vi "Fetch Multiple Record Multiple Channel (Wfm).vi"(5 "FIFO Type":T1=enum."Fast FIFO", 7 "Timeout (s)":i32=5, 8 "error in":errorcluster, 10 "Records to Fetch":i32, 11 "FPGA VI Reference In":refnum<k20>) -> (0 "error out":errorcluster, 2 "Acquired Data":waveform(dbl)[](array[waveform]), 3 "FPGA VI Reference Out":refnum<k20>, 4 "Elements Remaining":u32)   [LabVIEW 2012]
uses:
  <userlib>/FlexRIO Host Library/FlexRIO Host API/Acquire/FIFO Type.ctl
  <userlib>/FlexRIO Host Library/FlexRIO Host API/Acquire/Fetch/Fetch Acquired Data (I16).vi
  <vilib>/Utility/error.llb/Error Cluster From Error Code.vi
  <vilib>/rvi/errors/niLvFpgaAdjustHostInterfaceError.vi
  <vilib>/rvi/interface/nirviReadWriteControl/nirviReadWriteControl.xnode
  NiFpgaLv.dll
  <vilib>/rvi/interface/Simulation/niFpgaSimulationCallBeginRW.vi
  <userlib>/FlexRIO Host Library/FlexRIO Host Library (User).lvlib
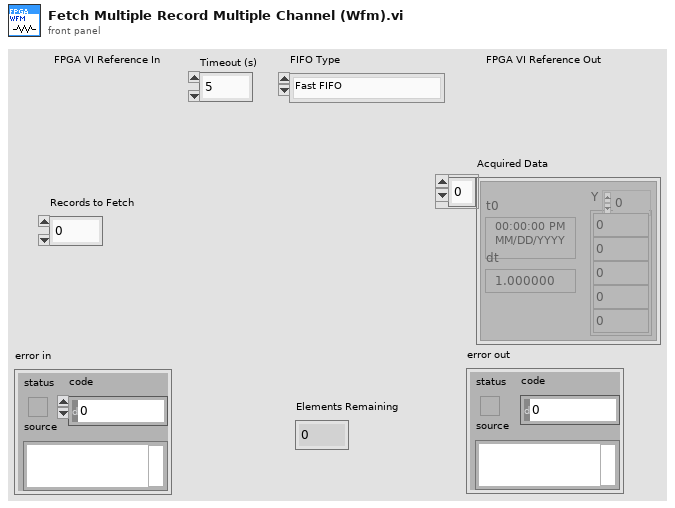
[diagram p1: front panel]
types:
  T1 = typedef "FIFO Type.ctl" = enum16{"FPGA to Host FIFO (U64)", "Generic", "FPGA to Host FIFO (U32)", "Fast FIFO"}
  T2 = cluster{"Load Record Parameters?":bool, "Pre Trigger Samples":u16, "Samples per Record":u16, "Trigger Hold Off":u16, "Record Count":u16}
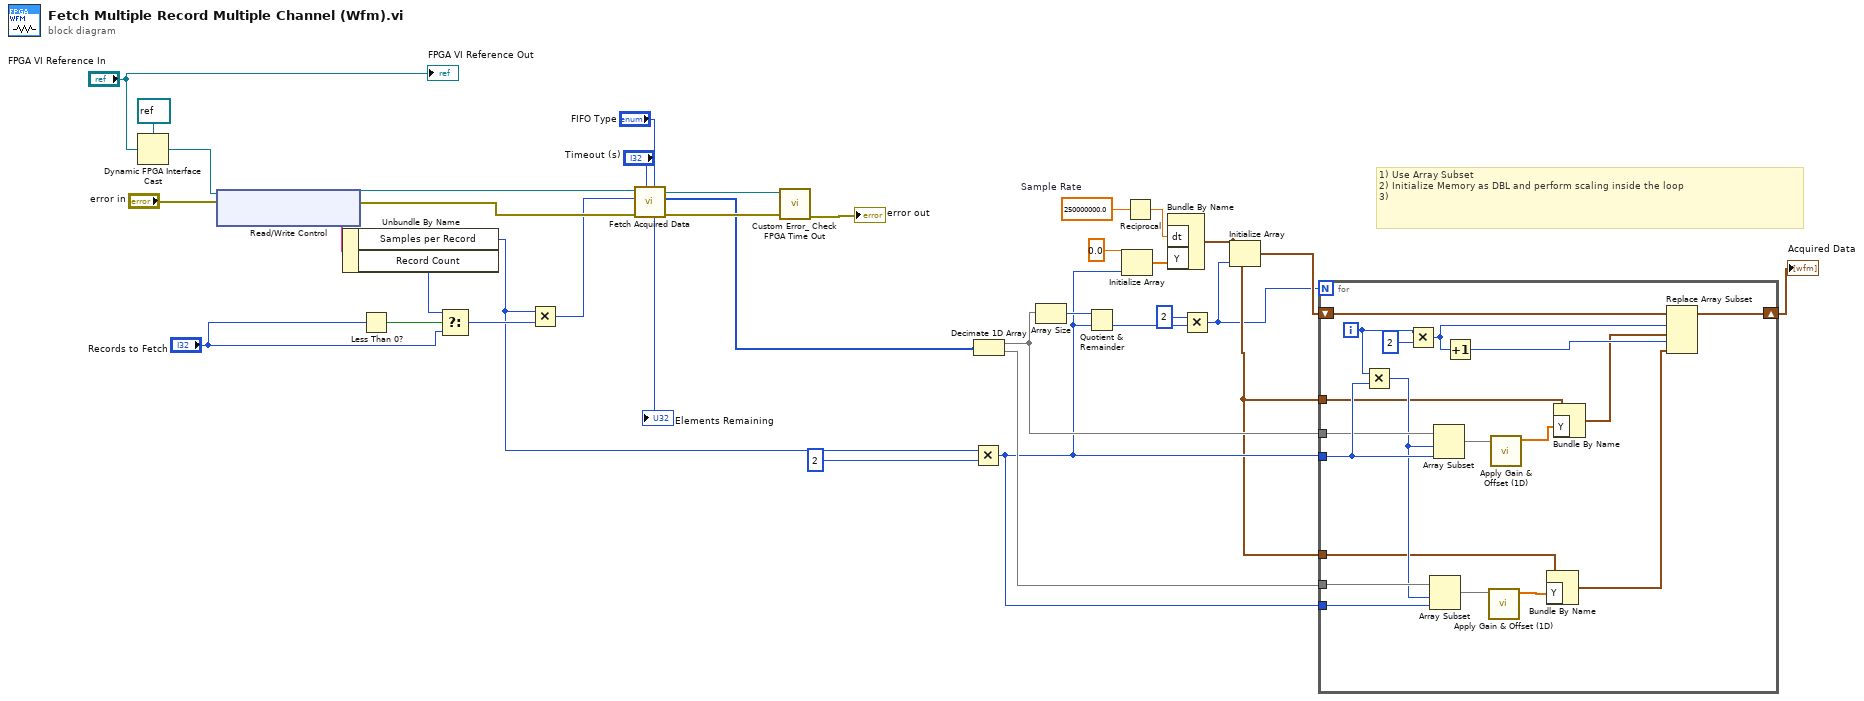
[diagram p0: block diagram]
diagram:
  w5 = 250000000.0  # Sample Rate
  # "1) Use Array Subset\n2) Initialize Memory as DBL and perform scaling inside the loop\n3)"
  n1 = Dynamic FPGA Interface Cast(Session In=refnum<k20> refnum ("Type"), Type="FPGA VI Reference In") -> (Session Out=w32:refnum<k20>)
  n2 = xnode "Read/Write Control"("FPGA VI Reference In"=w32, "error in"="error in") -> ("FPGA VI Reference Out"=w27:refnum<k20>, "error out"=w26:errorcluster, "Record Parameters"=w31:T2)
  n3 = Unbundle By Name(w31) -> ("Samples per Record"=w21:u16, "Record Count"=w29:u16)
  n4 = Less Than 0?(x="Records to Fetch") -> (x < 0?=w30:bool)
  n5 = Select(t=w29, s=w30, f="Records to Fetch") -> (s? t:f=w22:i32)
  n6 = Multiply(x=w21, y=w22) -> (x*y=w25:i32)
  n7 = call-poly <userlib>:"Fetch Acquired Data.vi"("FIFO Type"="FIFO Type", "Timeout (s)"="Timeout (s)", "error out"=w26, "Samples"=w25, "FPGA Reference In"=w27) -> ("error out"=w16:errorcluster, "Data"=w2:i16[], "FPGA Reference Out"=w17:refnum<k20>, "Elements Remaining"=→"Elements Remaining":u32)  [unwired: 3 in]
  n8 = call <userlib>:"Custom Error_ Check FPGA Time Out.vi"("error in"=w16, "FPGA VI Reference In"=w17) -> ("error out"=→"error out":errorcluster)  [unwired: 8 in, 1 out]
  n9 = Multiply(x=w21, y=u16 2) -> (x*y=w10:u16)
  n10 = Decimate 1D Array(w2) -> (w19:i16[], w12:i16[])
  n11 = Array Size(array=w19) -> (size(s)=w18:i32)
  n12 = Quotient & Remainder(x=w18, y=w10) -> (floor(x/y)=w14:i32)  [unwired: 1 out]
  n13 = Initialize Array(0.0 ("element"), w10) -> (w11:dbl[])
  n14 = Reciprocal(x=w5) -> (1/x=w4:dbl)
  n15 = Bundle By Name("dt"=w4, "Y"=w11) -> (w8:waveform(dbl))  [unwired: 1 in]
  n16 = Multiply(x=2, y=w14) -> (x*y=w6:i32)
  n17 = Initialize Array(w8, w6) -> (w9:waveform(dbl)[])
  n18 = for {
    N: w6 -> [_]
    tunnel: w19 -> [w53]
    tunnel: w10 -> [w54]
    tunnel: w12 -> [w52]
    tunnel: w10 -> [w50]
    shift-right: [w48] -> w7
    shift-left: w9 -> [w49]
    tunnel: w8 -> [w41]
    tunnel: w8 -> [w38]
    i -> [w45]
    n19 = Multiply(x=w45, y=w54) -> (x*y=w51:i32)
    n20 = Multiply(x=w45, y=2) -> (x*y=w43:i32)
    n21 = Array Subset(array=w52, index=w51, length=w50) -> (w46:i16[])
    n22 = Array Subset(array=w53, index=w51, length=w54) -> (w47:i16[])
    n23 = Increment(x=w43) -> (x+1=w42:i32)
    n24 = call <userlib>:"Apply Gain & Offset (1D).vi"("Raw Data"=w46) -> ("Scaled Data"=w39:dbl[])  [unwired: 10 in]
    n25 = call <userlib>:"Apply Gain & Offset (1D).vi"("Raw Data"=w47) -> ("Scaled Data"=w40:dbl[])  [unwired: 10 in]
    n26 = Bundle By Name(cluster=w38, "Y"=w39) -> (w36:waveform(dbl))
    n27 = Bundle By Name(cluster=w41, "Y"=w40) -> (w37:waveform(dbl))
    n28 = Replace Array Subset(array=w49, new element #1=w37, index #1=w43, new element #2=w36, index #2=w42) -> (w48:waveform(dbl)[])
  }
  "Acquired Data" <- w7
  "FPGA VI Reference Out" <- "FPGA VI Reference In"
